vi "Dynamic call-Calibration Toolbox Window.vi"(8 "error in (no error)":errorcluster) -> (0 "error out":errorcluster)   [LabVIEW 2020]
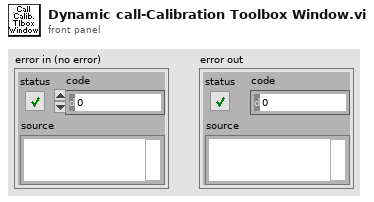
[diagram p1: front panel]
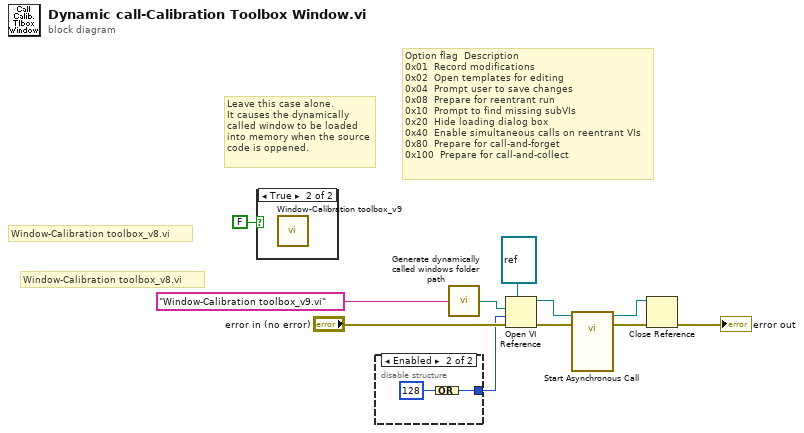
[diagram p0: block diagram]
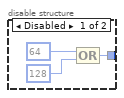
[diagram p2: hidden frame]
diagram:
  # "Window-Calibration toolbox_v8.vi"
  # "Window-Calibration toolbox_v8.vi"
  # "Leave this case alone.\nIt causes the dynamically called window to be loaded into memory when the source code is oppened."
  # "Option flag \tDescription\n0x01 \tRecord modifications\n0x02 \tOpen templates for editing\n0x04 \tPrompt user to save changes\n0x08 \tPrepare for reentrant run\n0x10 \tPrompt to find missing subVIs\n0x20 \tHide loading dialog box\n0x40 \tEnable simultaneous calls on reentrant VIs\n0x80 \tPrepare for call-and-forget\n0x100 \tPrepare for call-and-collect"
  n1 = case shown="True" FALSE {
    frame False {
    }
    frame True {
      n2 = call "Window-Calibration toolbox_v9.vi"() -> ()  [unwired: 12 in]
    }
  }
  n3 = disable-structure shown="Enabled" {
    disable-tunnel: [w14 w16] -> w4
    frame Disabled {
      n4 = Compound Arithmetic op=OR(64, 128) -> (w14:i32)
    }
    frame Enabled {
      n5 = Compound Arithmetic op=OR(128) -> (w16:i32)
    }
  }
  n6 = call "Generate dynamically called windows folder path.vi"("name of dynamically called VI"="Window-Calibration toolbox_v9.vi" ("Error Source")) -> ("Dynamically called VI path"=w7:path)
  n7 = Open VI Reference(type specifier VI Refnum (for type only)=refnum<vi> refnum, vi path=w7, options=w4, error in (no error)="error in (no error)") -> (vi reference=w5:refnum<vi>, error out=w6:errorcluster)  [unwired: 2 in]
  n8 = call-by-ref "Start Asynchronous Call"(reference=w5, error in=w6) -> (reference out=w1:refnum<vi>, error out=w2:errorcluster)  [unwired: 12 in]
  n9 = Close Reference(reference=w1, error in (no error)=w2) -> (error out=→"error out":errorcluster)
